vi "Sub Path Vars.vi"(8 "error in (no error)":errorcluster, 11 "path":path) -> (0 "error out":errorcluster, 3 "abs path":path)   [LabVIEW 2016]
doc: "Replaces path variables with their corresponding location on the file system. Supported path variables include %HOME%, %DOCS%, %DESKTOP%, %APPDATA%, and %TEMP%."
uses:
  <vilib>/Utility/sysdir.llb/System Directory Type.ctl
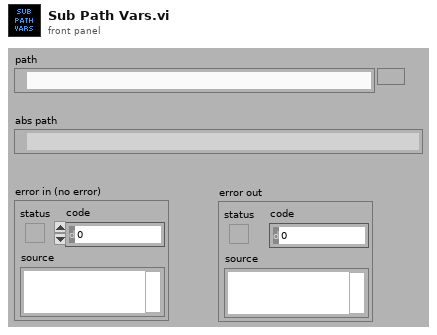
[diagram p1: front panel]
types:
  T1 = typedef "System Directory Type.ctl" = i32
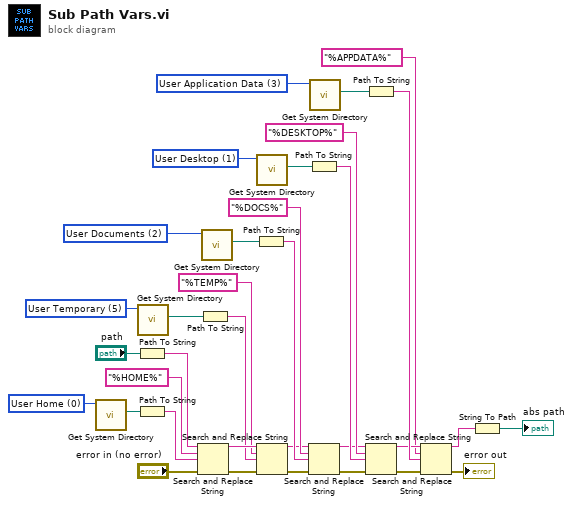
[diagram p0: block diagram]
diagram:
  w12 = T1 3 items=["User Home"=0, "User Desktop"=1, "User Documents"=2, "User Application Data"=3, "User Preferences"=4, "User Temporary"=5, "Public Documents"=6, "Public Application Data"=7, "Public Preferences"=8, "Public Cache"=13, "System Core Libraries"=9, "System Installed Libraries"=10, "Application Files"=11, "Boot Volume Root"=12] ("system directory type")
  w13 = T1 2 items=["User Home"=0, "User Desktop"=1, "User Documents"=2, "User Application Data"=3, "User Preferences"=4, "User Temporary"=5, "Public Documents"=6, "Public Application Data"=7, "Public Preferences"=8, "Public Cache"=13, "System Core Libraries"=9, "System Installed Libraries"=10, "Application Files"=11, "Boot Volume Root"=12] ("system directory type")
  w17 = T1 1 items=["User Home"=0, "User Desktop"=1, "User Documents"=2, "User Application Data"=3, "User Preferences"=4, "User Temporary"=5, "Public Documents"=6, "Public Application Data"=7, "Public Preferences"=8, "Public Cache"=13, "System Core Libraries"=9, "System Installed Libraries"=10, "Application Files"=11, "Boot Volume Root"=12] ("system directory type")
  w23 = T1 5 items=["User Home"=0, "User Desktop"=1, "User Documents"=2, "User Application Data"=3, "User Preferences"=4, "User Temporary"=5, "Public Documents"=6, "Public Application Data"=7, "Public Preferences"=8, "Public Cache"=13, "System Core Libraries"=9, "System Installed Libraries"=10, "Application Files"=11, "Boot Volume Root"=12] ("system directory type")
  w34 = T1 0 items=["User Home"=0, "User Desktop"=1, "User Documents"=2, "User Application Data"=3, "User Preferences"=4, "User Temporary"=5, "Public Documents"=6, "Public Application Data"=7, "Public Preferences"=8, "Public Cache"=13, "System Core Libraries"=9, "System Installed Libraries"=10, "Application Files"=11, "Boot Volume Root"=12] ("system directory type")
  n1 = call <vilib>:"Get System Directory.vi"("system directory type"=w34) -> ("system directory"=w32:path)  [unwired: 10 in]
  n2 = Path To String(path="path") -> (string=w30:string)
  n3 = Path To String(path=w32) -> (string=w33:string)
  n4 = call <vilib>:"Get System Directory.vi"("system directory type"=w23) -> ("system directory"=w24:path)  [unwired: 10 in]
  n5 = Search and Replace String(input string=w30, search string="%HOME%", replace string=w33, error in="error in (no error)") -> (result string=w27:string, error out=w28:errorcluster)  [unwired: 4 in, 2 out]
  n6 = Path To String(path=w24) -> (string=w25:string)
  n7 = call <vilib>:"Get System Directory.vi"("system directory type"=w13) -> ("system directory"=w14:path)  [unwired: 10 in]
  n8 = Path To String(path=w14) -> (string=w20:string)
  n9 = call <vilib>:"Get System Directory.vi"("system directory type"=w17) -> ("system directory"=w18:path)  [unwired: 10 in]
  n10 = Search and Replace String(input string=w27, search string="%TEMP%", replace string=w25, error in=w28) -> (result string=w4:string, error out=w22:errorcluster)  [unwired: 4 in, 2 out]
  n11 = Path To String(path=w18) -> (string=w19:string)
  n12 = Search and Replace String(input string=w4, search string="%DOCS%", replace string=w20, error in=w22) -> (result string=w3:string, error out=w21:errorcluster)  [unwired: 4 in, 2 out]
  n13 = call <vilib>:"Get System Directory.vi"("system directory type"=w12) -> ("system directory"=w11:path)  [unwired: 10 in]
  n14 = Path To String(path=w11) -> (string=w10:string)
  n15 = Search and Replace String(input string=w3, search string="%DESKTOP%", replace string=w19, error in=w21) -> (result string=w6:string, error out=w9:errorcluster)  [unwired: 4 in, 2 out]
  n16 = Search and Replace String(input string=w6, search string="%APPDATA%", replace string=w10, error in=w9) -> (result string=w8:string, error out=→"error out":errorcluster)  [unwired: 4 in, 2 out]
  n17 = String To Path(string=w8) -> (path=→"abs path":path)
